vi "Finalize.vi"(8 "error in":errorcluster, 11 "Plugin in":refnum<class "Output Sequencer.lvclass">) -> (0 "error out":errorcluster, 3 "Plugin out":refnum<class "Output Sequencer.lvclass">)   [LabVIEW 2024, in "Output Sequencer.lvlib" / "Output Sequencer.lvclass"]
uses:
  Output Sequencer.lvclass
  Types/UI Event.ctl
  Types/Event Type.ctl
  Output Sequencer.lvclass/Output Sequencer.ctl
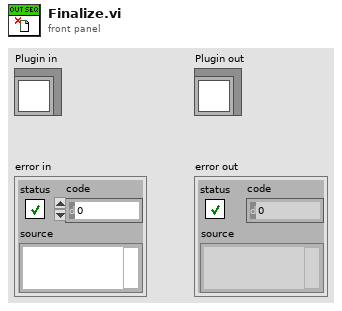
[diagram p1: front panel]
types:
  T1 = typedef "Output Sequencer.lvlib/Output Sequencer.lvclass/Event Type.ctl" = enum16{"Channel Update", "Test State Change", "Stop"}
  T2 = typedef "Output Sequencer.lvlib/Output Sequencer.lvclass/UI Event.ctl" = cluster{"Type":T1, "Data":variant}
  T3 = typedef "Output Sequencer.lvlib/Output Sequencer.lvclass/UI Ref.ctl" = refnum<vi>
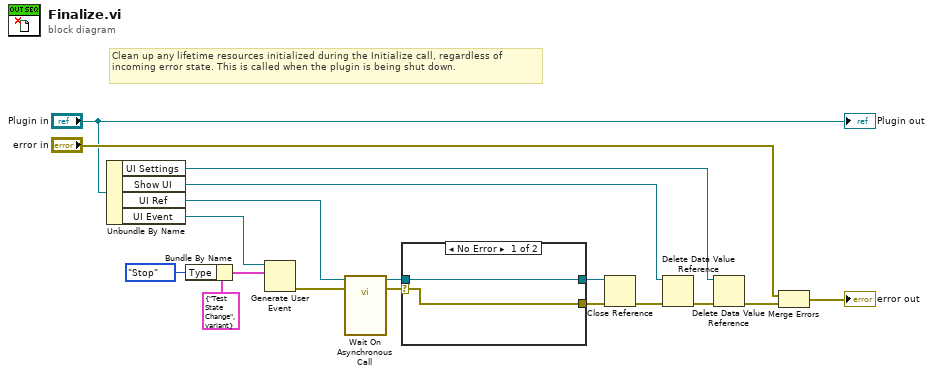
[diagram p0: block diagram]
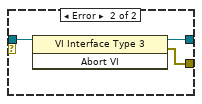
[diagram p2: hidden frame]
diagram:
  # "Clean up any lifetime resources initialized during the Initialize call, regardless of incoming error state. This is called when the plugin is being shut down."
  n1 = Unbundle By Name("Plugin in") -> ("UI Settings"=w2:refnum<data-value>, "Show UI"=w4:refnum<data-value>, "UI Ref"=w9:T3, "UI Event"=w12:refnum<user-event>)
  n2 = Bundle By Name(cluster=T2 {"Type"=enum."Test State Change", "Data"=variant} ("UI Event"), "Type"=Event_Type."Stop") -> (w15:T2)
  n3 = Generate User Event(user event=w12, event data cluster=w15) -> (error out=w6:errorcluster)  [unwired: 2 in, 1 out]
  n4 = call-by-ref "Wait On Asynchronous Call"(reference=w9, error in=w6) -> (reference out=w10:T3, error out=w11:errorcluster)  [unwired: 12 in]
  n5 = case shown="No Error" w11 {
    selector: w11 -> [w19 _]
    tunnel: w10 -> [w20 w23]
    tunnel: [w20 w22] -> w8
    tunnel: [w19 w21] -> w7
    frame No Error {
    }
    frame Error {
      n6 = invoke class="VI Interface Type 3" method="Abort VI"(reference=w23) -> (reference out=w22:T3, error out=w21:errorcluster)  [unwired: 2 in, 1 out]
    }
  }
  n7 = Close Reference(reference=w8, error in (no error)=w7) -> (error out=w5:errorcluster)
  n8 = Delete Data Value Reference(data value reference=w4, error in=w5) -> (error out=w3:errorcluster)  [unwired: 1 out]
  n9 = Delete Data Value Reference(data value reference=w2, error in=w3) -> (error out=w1:errorcluster)  [unwired: 1 out]
  n10 = Merge Errors("error in", w1) -> (→"error out":errorcluster)
  "Plugin out" <- "Plugin in"
